vi "cache tag indices.vi"(8 "error in":errorcluster, 9 "index cluster":variant, 10 "channel classification":T1, 11 "fixed channel runtime in":refnum<class "fixed channel runtime.lvclass">) -> (0 "error out":errorcluster, 3 "fixed channel runtime out":refnum<class "fixed channel runtime.lvclass">)   [LabVIEW 2013, in "fixed channel runtime.lvclass"]
uses:
  fixed channel runtime.lvclass
  <vilib>/NI/Tag Bus Module Framework/channel/channel classification.ctl
  <vilib>/NI/Tag Bus Module Framework/channel/TBM channel.lvclass
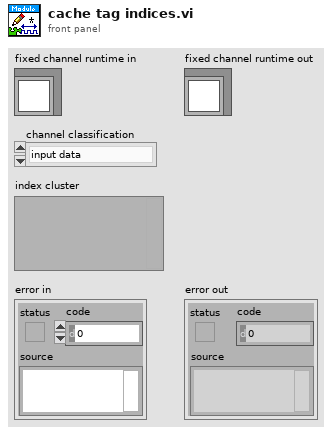
[diagram p1: front panel]
types:
  T1 = typedef "TBM channel.lvclass/channel classification.ctl" = enum16{"input data", "output data", "processing parameter", "processing result"}
  T2 = typedef "fixed channel configuration.lvclass/index type definitions.ctl" = cluster{"input indices":variant, "parameter indices":variant, "result indices":variant, "output indices":variant}
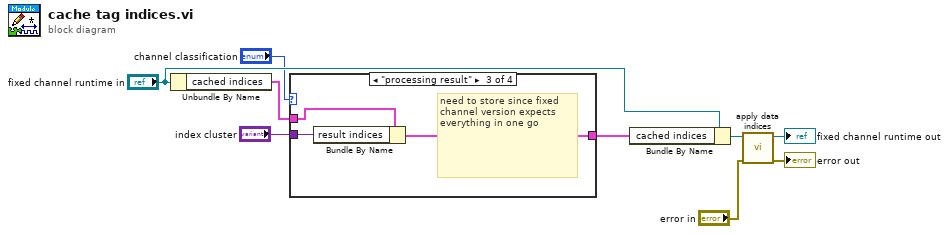
[diagram p0: block diagram]
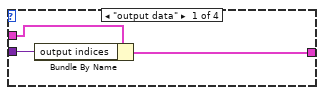
[diagram p2: hidden frame]
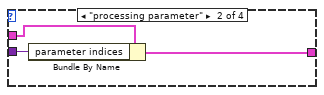
[diagram p3: hidden frame]
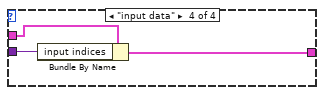
[diagram p4: hidden frame]
diagram:
  n1 = Unbundle By Name("fixed channel runtime in") -> ("cached indices"=w2:T2)
  n2 = case shown="\"processing result\"" "channel classification" {
    tunnel: [w11 w14 w17 w20] -> w3
    tunnel: w2 -> [w12 w15 w18 w21]
    tunnel: "index cluster" -> [w10 w13 w16 w19]
    frame "output data" {
      n3 = Bundle By Name(cluster=w12, "output indices"=w10) -> (w11:T2)
    }
    frame "processing parameter" {
      n4 = Bundle By Name(cluster=w15, "parameter indices"=w13) -> (w14:T2)
    }
    frame "processing result" {
      # "need to store since fixed channel version expects everything in one go"
      n5 = Bundle By Name(cluster=w18, "result indices"=w16) -> (w17:T2)
    }
    frame "input data" {
      n6 = Bundle By Name(cluster=w21, "input indices"=w19) -> (w20:T2)
    }
  }
  n7 = Bundle By Name(cluster="fixed channel runtime in", "cached indices"=w3) -> (w5:refnum<class "fixed channel runtime.lvclass">)
  n8 = call-dynamic "apply data indices.vi"("error in"="error in", "fixed channel runtime in"=w5) -> ("error out"=→"error out":errorcluster, "fixed channel runtime out"=→"fixed channel runtime out":refnum<class "fixed channel runtime.lvclass">)  [unwired: 8 in]
